vi "c.vi"() -> (4 "移動單位":cluster{"移動單位":dbl, "自轉單位":dbl})   [LabVIEW 2019]
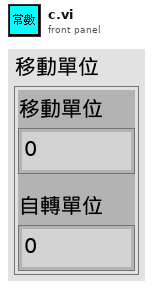
[diagram p1: front panel]
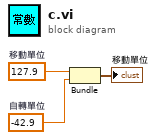
[diagram p0: block diagram]
diagram:
  w2 = -42.9  # 自轉單位
  w3 = 127.9  # 移動單位
  n1 = Bundle("移動單位"=w3, "自轉單位"=w2) -> (→"移動單位":cluster{"移動單位":dbl, "自轉單位":dbl})  [unwired: 1 in]
